vi "Change Glyphs Snippet.vi"(11 "引用":refnum<vi>) -> ()   [LabVIEW 2017, in "Tree API.lvlib" / "Tree.lvclass"]
doc: "Recursively traverse down wired Tree ID and populate the Tree Control with the contents of the Tree.\n\nBecause the Tree Control requires to have only one root element, the Root ID has to be specified. This means that if you have multiple roots in your Tree you need to visualize them seperately."
uses:
  Tree.lvclass
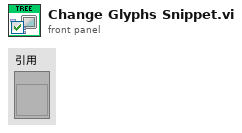
[diagram p1: front panel]
types:
  T1 = cluster{"Left Cell String":string, "Child Text":string[], "Child Tag":string, "Item Indent":i32, "Child Only?":bool, "Glyph Index":i32}[]
  T2 = cluster{"Left Cell String":string, "Child Text":string[], "Child Tag":string, "Item Indent":i32, "Child Only?":bool, "Glyph Index":i32}
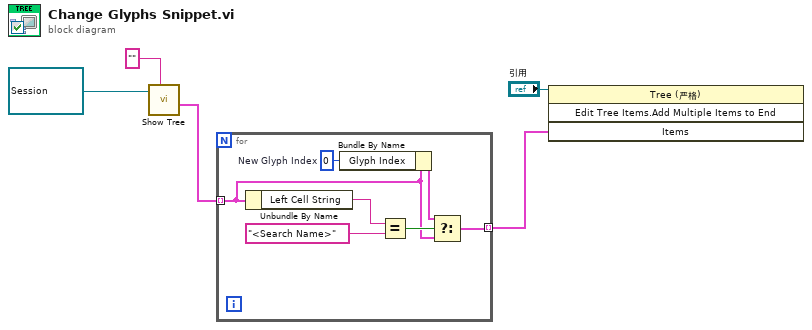
[diagram p0: block diagram]
diagram:
  n1 = call "Show Tree.vi"("Root ID"="", "Tree"=refnum<data-value> refnum) -> ("Items Out"=w3:T1)  [unwired: 7 in, 2 out]
  n2 = for {
    tunnel: w3 -> [w8] mode=indexing
    tunnel: [w6] -> w2 mode=indexing
    w7 = 0  # New Glyph Index
    n3 = Unbundle By Name(w8) -> ("Left Cell String"=w12:string)
    n4 = Bundle By Name(cluster=w8, "Glyph Index"=w7) -> (w9:T2)
    n5 = Equal?(x=w12, y="<Search Name>") -> (x = y?=w11:bool)
    n6 = Select(t=w9, s=w11, f=w8) -> (s? t:f=w6:T2)
  }
  n7 = invoke class="Tree (严格)" method="Edit Tree Items.Add Multiple Items to End"(reference="引用", "Items"=w2) -> ()  [unwired: 2 in, 4 out]
